vi "SetExtTrig.vi"(1 "boards":u32) -> ()   [LabVIEW 2015]
uses:
  ESLSCDLL.dll
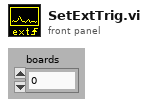
[diagram p1: front panel]
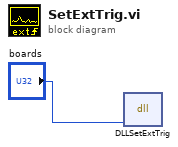
[diagram p0: block diagram]
diagram:
  n1 = dll-call lib="C:/ENTW/PCIE/64bit/lv64/lv64/board.vis/ESLSCDLL.dll" fn="DLLSetExtTrig"("drv"="boards") -> ()  [unwired: 5 in, 2 out]
